vi "nominal run end.vi"(8 "error in (no error)":errorcluster, 9 "is_present":bool, 10 "out_millis":dbl, 11 "run":i32) -> (0 "error out":errorcluster, 1 "is_present out":bool, 2 "out_millis out":dbl, 3 "function return":i32)   [LabVIEW 2020, in "client.lvlib"]
doc: "int32_t nominal_run_end(int32_t run, double *out_millis, bool *is_present);"
uses:
  client.lvlib
  bin/nominalClient_64.dll
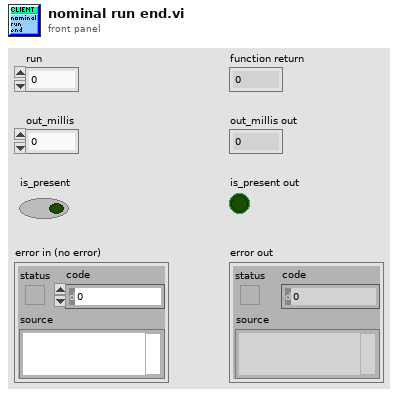
[diagram p1: front panel]
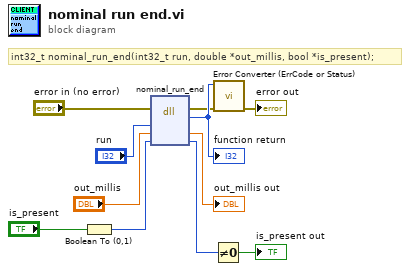
[diagram p0: block diagram]
diagram:
  # "int32_t nominal_run_end(int32_t run, double *out_millis, bool *is_present);"
  n1 = Boolean To (0,1)(Boolean="is_present") -> (0, 1=w6:i16)
  n2 = dll-call lib="C:/code/labview-client-rs/lv_src/bin/nominalClient_*.*" fn="nominal_run_end"(error in="error in (no error)", "run"="run", "out_millis"="out_millis", "is_present"=w6) -> (error out=w2:errorcluster, w11:i32, "out_millis"=→"out_millis out":dbl, "is_present"=w4:u8)  [unwired: 3 in, 1 out]
  "function return" <- w11
  n3 = Not Equal To 0?(x=w4) -> (x != 0?=→"is_present out":bool)
  n4 = call "Error Converter (ErrCode or Status).vi"("error in (no error)"=w2, "error code"=w11) -> ("error out"=→"error out":errorcluster)  [unwired: 9 in]
